vi "Use Adaptive Filter (Array).vi"() -> ()   [LabVIEW 2019]
doc: "This example demonstrates how to create and use an adaptive filter. This example simulates and filters signals in block-by-block mode.\n\nComplete the following steps to use this example.\n\n1. Run this VI. Observe how the coefficients of the adaptive filter converge to those of the unknown system.\n\n2. Browse the block diagram of this example to understand how this example uses the adaptive filter VIs.\n\n3. Replace the AFT Create FIR LMS VI with other filter creation VIs palette to try other adaptive filter algorithms.\n\nThis example uses an FIR LMS adaptive filter to identify the impulse response of an unknown system. A lowpass FIR filter simulates the unknown system. The input to both this system and the adaptive filter is Gaussian white noise. The output of this system is the reference of the adaptive filter."
uses:
  <vilib>/addons/Adaptive Filters/Create/AFT Create FIR LMS (Real).vi
  <vilib>/addons/Adaptive Filters/Processing/AFT Filter Signal and Update Coefficients (Real, Array).vi
  <vilib>/addons/Adaptive Filters/Analysis/AFT Get Coefficients (FIR, Real).vi
  <vilib>/addons/Adaptive Filters/NI_AdaptiveFilter.lvlib
panel:
  in  "Stop":bool
  in  "Step Size":dbl=0.002 min=0.0 step=0.001
  in  "Filter Length":i32=25 min=2
  out "Coefficients":dbl[][](graph)
  out "Error Signal":dbl[](graph)
  # "Select Help>>Show Context Help and move the cursor over the VI icon of this example for more information."
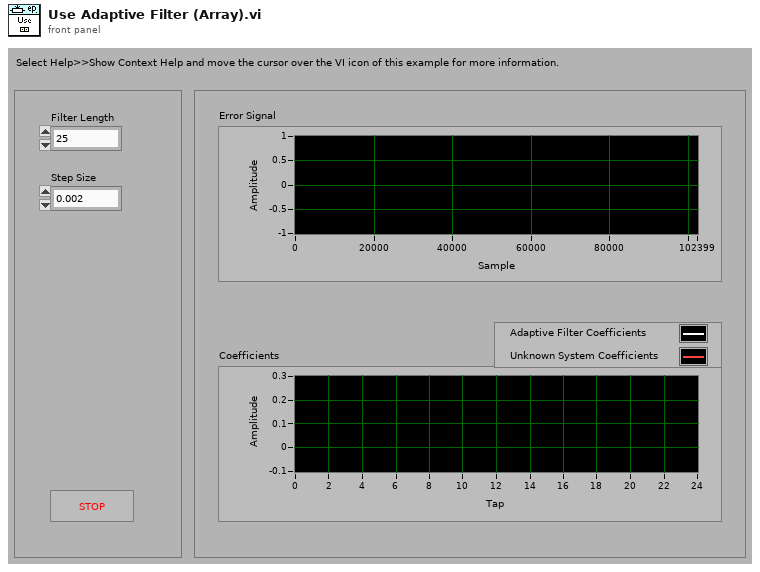
[diagram p1: front panel]
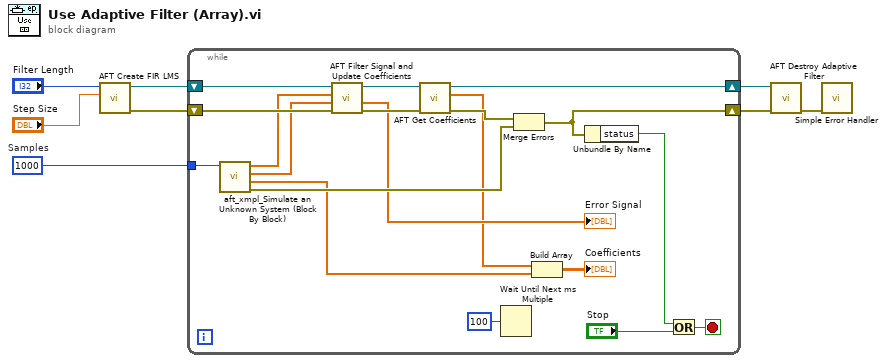
[diagram p0: block diagram]
diagram:
  w4 = 1000  # Samples
  n1 = call-poly <vilib>:"AFT Create FIR LMS.vi"("step size"="Step Size", "filter length"="Filter Length") -> ("error out"=w6:errorcluster, "adaptive filter out"=w7:refnum<k20>)  [unwired: 2 in, 6 out]
  n2 = while {
    tunnel: w4 -> [w16]
    shift-right: [w14] -> w3
    shift-left: w7 -> [w25]
    shift-right: [w10] -> w2
    shift-left: w6 -> [w24]
    stop <- w11 stop-if-true
    n3 = call "aft_xmpl_Simulate an Unknown System (Block By Block).vi"("samples"=w16) -> ("error out"=w26:errorcluster, "unknown system coefficients"=w15:dbl[], "response signal"=w17:dbl[], "stimulus signal"=w18:dbl[])  [unwired: 4 in, 3 out]
    n4 = call-poly <vilib>:"AFT Filter Signal and Update Coefficients.vi"("error in (no error)"=w24, "d(n)"=w17, "x(n)"=w18, "adaptive filter in"=w25) -> ("error out"=w22:errorcluster, "e(n)"=→"Error Signal":dbl[], "adaptive filter out"=w23:refnum<k20>)  [unwired: 2 in, 3 out]
    n5 = call-poly <vilib>:"AFT Get Coefficients.vi"("error in (no error)"=w22, "adaptive filter in"=w23) -> ("error out"=w27:errorcluster, "coefficients"=w20:dbl[], "adaptive filter out"=w14:refnum<k20>)  [unwired: 7 out]
    n6 = Wait Until Next ms Multiple(millisecond multiple=u32 100) -> ()  [unwired: 1 out]
    n7 = Merge Errors(w27, w26) -> (w10:errorcluster)
    n8 = Build Array(w20, w15) -> (→"Coefficients":dbl[][])
    n9 = Unbundle By Name(w10) -> ("status"=w9:bool)
    n10 = Or(x=w9, y="Stop") -> (x .or. y?=w11:bool)
  }
  n11 = call <vilib>:"AFT Destroy Adaptive Filter.vi"("error in (no error)"=w2, "adaptive filter in"=w3) -> ("error out"=w1:errorcluster)  [unwired: 9 out]
  n12 = call <vilib>:"Simple Error Handler.vi"("error in (no error)"=w1) -> ()  [unwired: 1 in, 8 out]
